vi "ConnectToRobot.vi"(9 "ip":string, 10 "error in (no error)":errorcluster) -> (0 "HighSpeedEServer":refnum<k24>, 3 "error out":errorcluster)   [LabVIEW 2013, in "UnderAutomation.Yaskawa.lvlib"]
uses:
  UnderAutomation.Yaskawa.lvlib
  C:/Users/fg/Documents/Yaskawa.vi/LabVIEW_2024/UnderAutomation.Yaskawa/lib/UnderAutomation.Yaskawa.dll
  LabVIEW_2024/UnderAutomation.Yaskawa/lib/UnderAutomation.Yaskawa.dll
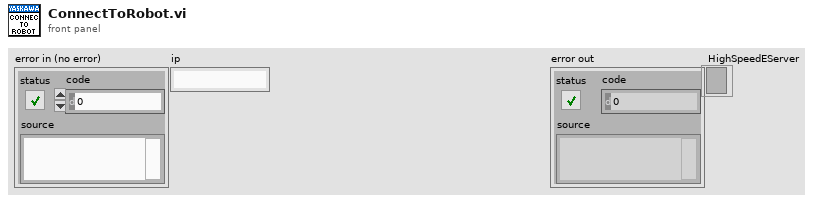
[diagram p1: front panel]
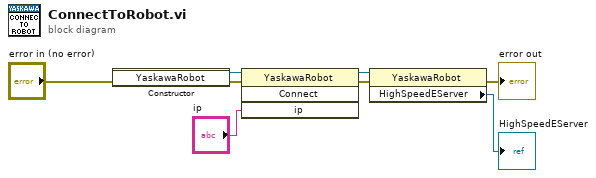
[diagram p0: block diagram]
diagram:
  n1 = constructor class="YaskawaRobot"(error in="error in (no error)") -> (reference out=w5:refnum<k24>, error out=w3:errorcluster)  [unwired: 2 in, 1 out]
  n2 = invoke class="YaskawaRobot" method="Connect"(reference=w5, error in=w3, "ip"="ip") -> (reference out=w4:refnum<k24>, error out=w2:errorcluster)  [unwired: 1 in, 2 out]
  n3 = property class="YaskawaRobot"(reference=w4, error in=w2) -> (error out=→"error out":errorcluster, "HighSpeedEServer"=→"HighSpeedEServer":refnum<k24>)  [unwired: 1 out]
